vi "FlatToRichhwval_GenericRequest.vi"(5 "OutputClusterType":T1, 11 "InputCluster":T2) -> (3 "OutputCluster":T1)   [LabVIEW 2025, in "Automotive-Vision-OOBService_client.lvlib"]
uses:
  hwval_GenericRequest_Flat.ctl
  hwval_GenericRequest.ctl
  Automotive-Vision-OOBService_client.lvlib
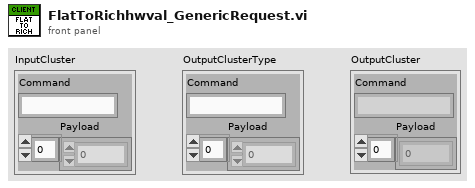
[diagram p1: front panel]
types:
  T1 = typedef "Automotive-Vision-OOBService_client.lvlib/hwval_GenericRequest.ctl" = cluster{"Command":string, "Payload":u8[]}
  T2 = typedef "Automotive-Vision-OOBService_client.lvlib/hwval_GenericRequest_Flat.ctl" = cluster{"Command":string, "Payload":u8[]}
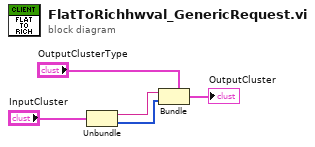
[diagram p0: block diagram]
diagram:
  n1 = Unbundle "Unbundle"("InputCluster") -> ("Command"=w2:string, "Payload"=w1:u8[])
  n2 = Bundle "Bundle"(cluster="OutputClusterType", "Command"=w2, "Payload"=w1) -> (→"OutputCluster":T1)
